vi "whichPmt.vi"(10 "element":u32 format="%032b") -> (1 "elementOut":u32 format="%032b", 2 "pmtNumber":u32)   [LabVIEW 2014]
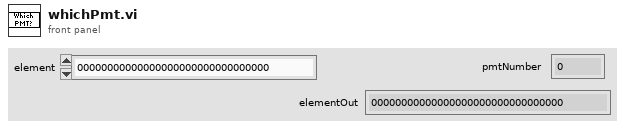
[diagram p1: front panel]
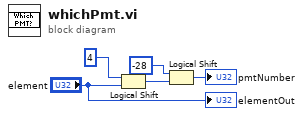
[diagram p0: block diagram]
diagram:
  n1 = Logical Shift(y=i16 4, x="element") -> (x << y=w3:u32)
  n2 = Logical Shift(y=i16 -28, x=w3) -> (x << y=→"pmtNumber":u32)
  "elementOut" <- "element"
